vi "SetFrameRate.vi"(8 "error in (no error)":errorcluster, 10 "Frame Rate":u8, 11 "CameraTestingProxyAPI in":refnum<class "CameraTestingProxyAPI.lvclass">) -> (0 "error out":errorcluster, 3 "CameraTestingProxyAPI out":refnum<class "CameraTestingProxyAPI.lvclass">)   [LabVIEW 2020, in "CameraTestingProxy.lvlib" / "CameraTestingProxyAPI.lvclass"]
uses:
  CameraTestingProxyAPI.lvclass
  7e2a72aa-0513-407a-a3b8-e21cf586ad4e.vi
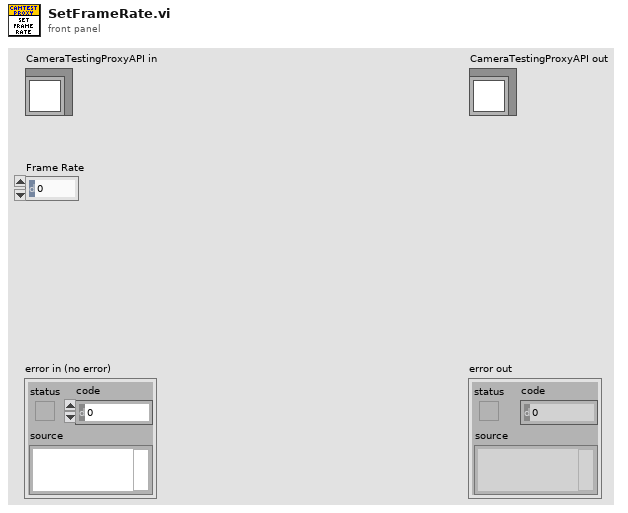
[diagram p1: front panel]
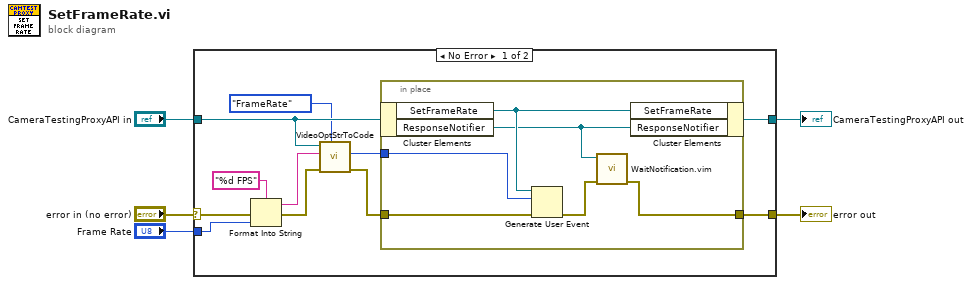
[diagram p0: block diagram]
diagram:
  n1 = case shown="No Error" "error in (no error)" {
    selector: "error in (no error)" -> [w9 w24]
    tunnel: "CameraTestingProxyAPI in" -> [w14 w23]
    tunnel: "Frame Rate" -> [w12 _]
    tunnel: [w16 w24] -> w2
    tunnel: [w15 w23] -> w1
    frame No Error {
      n2 = Format Into String(format string="%d FPS", error in=w9, w12) -> (resulting string=w10:string, error out=w8:errorcluster)  [unwired: 1 in]
      n3 = call "VideoOptStrToCode.vi"("VideoOption"=enum16{"FrameRate", "ImageType", "Resolution"}."FrameRate", "error in (no error)"=w8, "DescriptionString"=w10, "CameraTestingProxyAPI in"=w14) -> ("error out"=w7:errorcluster, "Code"=w13:u8)  [unwired: 5 in, 1 out]
      n4 = in-place {
        in-place-border: w7 -> [w22]
        in-place-border: [w18] -> w16
        in-place-border: w13 -> [w20]
        n5 = in-place-cluster #1(w14) -> ("SetFrameRate"=w21:refnum<user-event>, "ResponseNotifier"=w17:refnum<notifier>)
        n6 = Generate User Event(user event=w21, event data cluster=w20, error in=w22) -> (error out=w19:errorcluster)  [unwired: 1 in, 1 out]
        n7 = call "WaitNotification.vim"("error in (no error)"=w19, "ResponseNotifier"=w17) -> ("error out"=w18:errorcluster)  [unwired: 8 in, 1 out]
        n8 = in-place-cluster #1("SetFrameRate"=w21, "ResponseNotifier"=w17) -> (w15:refnum<class "CameraTestingProxyAPI.lvclass">)
      }
    }
    frame Error {
    }
  }
  "error out" <- w2
  "CameraTestingProxyAPI out" <- w1
